vi "Parse BTI ARINC 429 Record.vi"(11 "record":T3 {"type" format="%04x"; "timestamp" format="%08x"; "msgact" format="%04x"; "data" format="%08x"; "timestamph" format="%08x"}) -> (0 "receiving error":bool, 1 "hit":bool, 2 "time stamp":dbl, 3 "data word":u32 format="%032b", 4 "specific errors":T2, 5 "message info":T1)   [LabVIEW 2020, in "Ballard ARINC 429 Engine.lvlib" / "Custom Device.lvlib"]
uses:
  Custom Device.lvlib
  <instrlib>/BTICardLib/Public/Controls/429 Record.ctl
  <instrlib>/BTICardLib/BTICardLV.lvlib
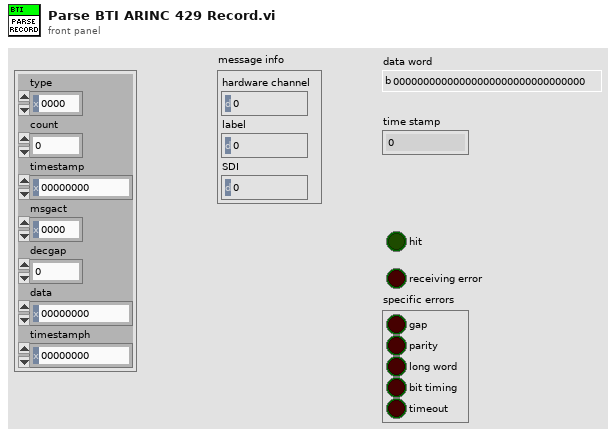
[diagram p1: front panel]
types:
  T1 = cluster{"hardware channel":u8, "label":u8, "SDI":u8}
  T2 = cluster{"gap":bool, "parity":bool, "long word":bool, "bit timing":bool, "timeout":bool}
  T3 = typedef "BTICardLV.lvlib/429 Record.ctl" = cluster{"type":u16, "count":u16, "timestamp":u32, "msgact":u16, "decgap":u16, "data":u32, "timestamph":u32}
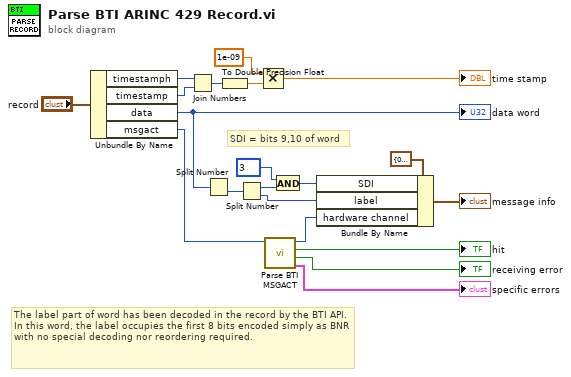
[diagram p0: block diagram]
diagram:
  # "SDI = bits 9,10 of word"
  # "The label part of word has been decoded in the record by the BTI API. In this word, the label occupies the first 8 bits encoded simply as BNR with no special decoding nor reordering required."
  n1 = Unbundle By Name("record") -> ("timestamph"=w14:u32, "timestamp"=w13:u32, "data"=w4:u32, "msgact"=w19:u16)
  "data word" <- w4
  n2 = Join Numbers(hi=w14, lo=w13) -> ((hi.lo)=w15:u64)
  n3 = Split Number(x=w4) -> (lo(x)=w9:u16)  [unwired: 1 out]
  n4 = To Double Precision Float(number=w15) -> (double precision float=w17:dbl)
  n5 = Split Number(x=w9) -> (hi(x)=w10:u8, lo(x)=w3:u8)
  n6 = Multiply(x=1e-09 ("y"), y=w17) -> (x*y=→"time stamp":dbl)
  n7 = call "Parse BTI MSGACT.vi"("msgact"=w19) -> ("specific errors"=→"specific errors":T2, "receiving error"=→"receiving error":bool, "hit"=→"hit":bool, "hardware channel"=w5:u8)  [unwired: 6 in, 1 out]
  n8 = And(x=u8 3, y=w10) -> (x .and. y?=w6:u8)
  n9 = Bundle By Name(cluster=T1 {"hardware channel"=0, "label"=0, "SDI"=0} ("message info"), "SDI"=w6, "label"=w3, "hardware channel"=w5) -> (→"message info":T1)
